vi "flattenData.vi"(11 "input array":dbl[](array[numeric])) -> (1 "flattened graph":dbl[](graph), 2 "flattned array":dbl[](array[numeric]))   [LabVIEW 2013]
uses:
  <vilib>/imath/engines/lvmath/Plug In/_Char/NIMS_CH_character datatype.ctl
  <vilib>/imath/engines/lvmath2/RunTimeEngine/BuiltInFunctions/double/NIMS_double.vi
  <instcachedir>/0/NIMS_double_34E32F64C2B04A25A042F4CA881A0A41.lvgen/NIMS_double_34E32F64C2B04A25A042F4CA881A0A41_003.vi
  <vilib>/imath/engines/lvmath2/RunTimeEngine/NodeEndStatement/NIMS_NodeEndStatement_Output.vi
  <instcachedir>/0/NIMS_NodeEndStatement_Output_53EC0D466D134D7ABD903AC30B43404B.lvgen/NIMS_NodeEndStatement_Output_53EC0D466D134D7ABD903AC30B43404B_001.vi
  <vilib>/imath/engines/lvmath2/RunTimeEngine/ErrorHandling/NIMS_Finalize Error.vi
  <vilib>/Analysis/NI_AALPro.lvlib
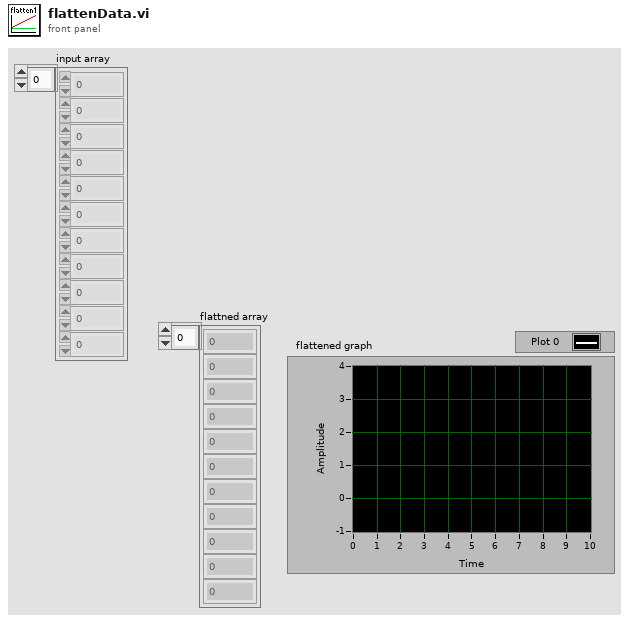
[diagram p1: front panel]
types:
  T1 = typedef "NIMS_CH_character datatype.ctl" = cluster{"Numeric":u8}
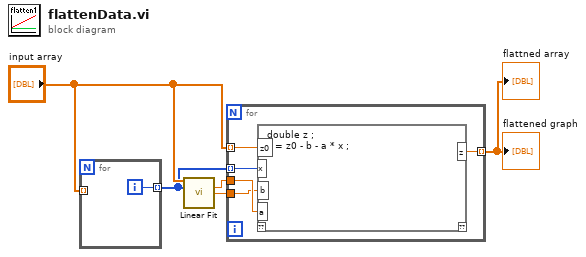
[diagram p0: block diagram]
diagram:
  n1 = for {
    tunnel: "input array" -> [_] mode=indexing
    tunnel: [w6] -> w1 mode=indexing
    i -> [w6]
  }
  n2 = call <vilib>:"Linear Fit.vi"("Y"="input array", "X"=w1) -> ("slope"=w2:dbl, "intercept"=w3:dbl)  [unwired: 9 in, 3 out]
  n3 = for {
    tunnel: "input array" -> [w11] mode=indexing
    tunnel: w1 -> [w10] mode=indexing
    tunnel: w2 -> [w9]
    tunnel: w3 -> [w8]
    tunnel: [w7] -> w5 mode=indexing
    n4 = mathscript code="double z ;\nz = z0 - b - a * x ;"("z0"=w11, "x"=w10, "b"=w8, "a"=w9) -> ("z"=w7:dbl)  [unwired: 1 in, 1 out]
  }
  "flattened graph" <- w5
  "flattned array" <- w5
